vi "WriteConfigClusterComplex.vi"(3 "error in (no error)":errorcluster, 4 "Cluster":refnum<vi>, 5 "Configfile input":T1) -> (0 "error out":errorcluster, 2 "refnum out":T1)   [LabVIEW 2009]
uses:
  <vilib>/Utility/config.llb/Config Data RefNum.ctl
  Write Key (String).vi
  <vilib>/Utility/config.llb/NI_LVConfig.lvlib
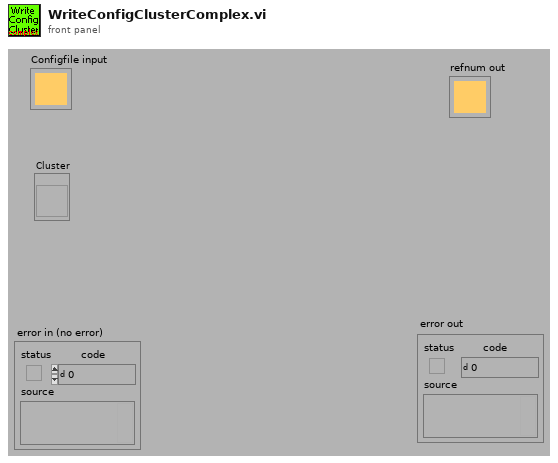
[diagram p1: front panel]
types:
  T1 = typedef "NI_LVConfig.lvlib/Config Data RefNum.ctl" = refnum<k1>
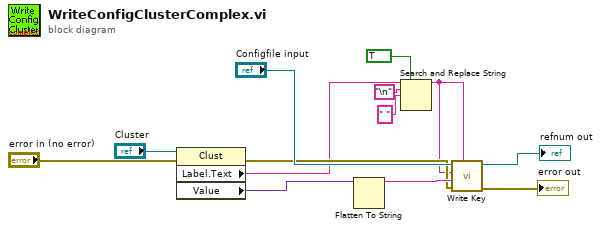
[diagram p0: block diagram]
diagram:
  n1 = property class="Clust"(reference="Cluster", error in="error in (no error)") -> (error out=w9:errorcluster, "Label.Text"=w6:string, "Value"=w12:variant)  [unwired: 1 out]
  n2 = Flatten To String(anything=w12) -> (data string=w11:string)  [unwired: 3 in, 2 out]
  n3 = Search and Replace String(replace all?=TRUE ("replace all? (F)"), input string=w6, search string="\n", replace string=" " ("replace string (\"\")")) -> (result string=w4:string)  [unwired: 4 in, 3 out]
  n4 = call-poly "Write Key.vi"("section"=w4, "error in (no error)"=w9, "value"=w11, "key"=w4, "refnum"="Configfile input") -> ("error out"=→"error out":errorcluster, "refnum out"=→"refnum out":T1)  [unwired: 5 in]
